vi "Get Available Components.vi"(8 "error in (no error)":errorcluster, 10 "Item Types (all visible)":T3 items=["all visible", "all including hidden", "standard only", "startup only"], 11 "Session in":refnum<k21>) -> (0 "error out":errorcluster, 2 "Software Components":T1[](array[typedef]) {"component type" items=["standard", "hidden", "system", "unknown", "startup", "image"]}, 3 "Session out":refnum<k21>)   [LabVIEW 2012, in "nisyscfg.lvlib"]
doc: "Retrieves a list of software components on the local system that are available for installation to the specified target."
uses:
  <vilib>/nisyscfg/nisyscfg.lvlib
  <vilib>/nisyscfg/Component Types.ctl
  <vilib>/nisyscfg/Software 1.2.ctl
  <vilib>/nisyscfg/Component Type.ctl
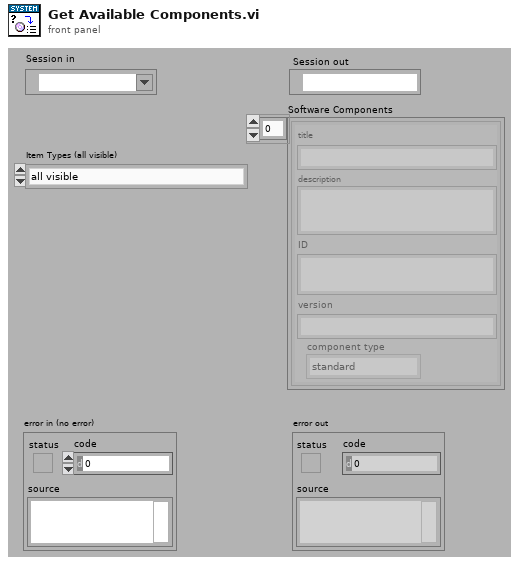
[diagram p1: front panel]
types:
  T1 = typedef "nisyscfg.lvlib/Software 1.2.ctl" = cluster{"title":string, "description":string, "ID":string, "version":string, "component type":T2}
  T2 = typedef "nisyscfg.lvlib/Component Type.ctl" = u32
  T3 = typedef "nisyscfg.lvlib/Component Types.ctl" = u32
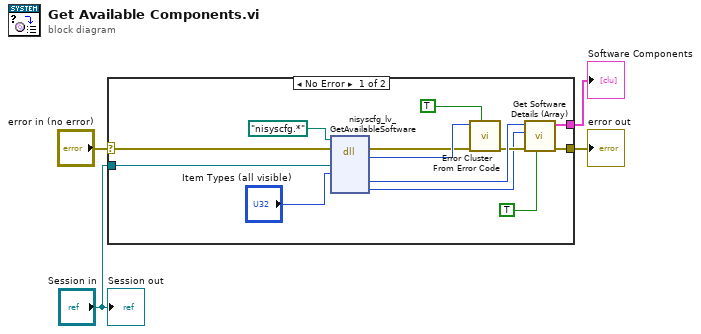
[diagram p0: block diagram]
diagram:
  n1 = case shown="No Error" "error in (no error)" {
    selector: "error in (no error)" -> [w15 w18]
    tunnel: [w9 w18] -> w4
    tunnel: "Session in" -> [w14 _]
    tunnel: [w8 _] -> w1
    frame No Error {
      n2 = dll-call lib="nisyscfg.*" fn="nisyscfg_lv_GetAvailableSoftware" label="GetAvailableSoftware"(path in=path "nisyscfg.*", error in=w15, "system"=w14, "includeTypes"="Item Types (all visible)") -> (error out=w16:errorcluster, "result"=w17:i32, "components"=w11:u64, "numComponents"=w7:i32)  [unwired: 5 in, 1 out]
      n3 = call <vilib>:"Error Cluster From Error Code.vi"("show call chain? (False)"=TRUE, "error in (no error)"=w16, "error code (0)"=w17) -> ("error out"=w10:errorcluster)  [unwired: 6 in]
      n4 = call <vilib>:"Get Software Details (Array).vi"("Trace Component Info (F)"=TRUE ("log to NI Spy (F)"), "error in (no error)"=w10, "Number of Elements"=w7, "Enumerator in"=w11) -> ("error out"=w9:errorcluster, "Software Components"=w8:T1[])  [unwired: 6 in]
    }
    frame Error {
    }
  }
  "error out" <- w4
  "Software Components" <- w1
  "Session out" <- "Session in"
